vi "u(t)L_test_7.vi"(6 "enable":bool, 7 "Desire Velosity":dbl(slide) scale=-10.0..10.0, 8 "Kd":dbl, 9 "Ki":dbl, 10 "Kp":dbl, 11 "Velocity":dbl) -> (2 "u(t)":dbl)   [LabVIEW 2018]
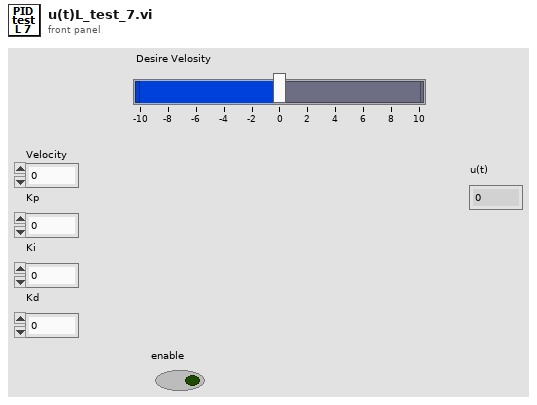
[diagram p1: front panel]
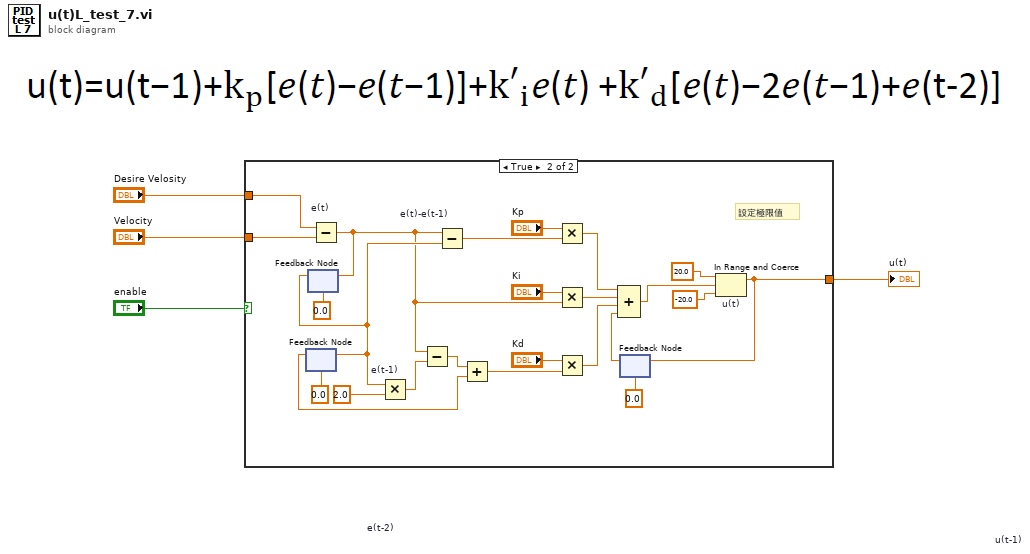
[diagram p0: block diagram]
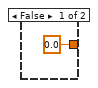
[diagram p2: hidden frame]
diagram:
  n1 = case shown="True" "enable" {
    tunnel: [0.0 ("upper limit") w29] -> w4
    tunnel: "Velocity" -> [_ w11]
    tunnel: "Desire Velosity" -> [_ w10]
    frame False {
    }
    frame True {
      # "設定極限值"
      n2 = feedback #1 "e(t-2)"(0.0) -> (w20:dbl)
      n3 = feedback #2 "e(t-1)"(0.0) -> (w9:dbl)
      n4 = feedback-in #1(w9) -> ()
      n5 = Subtract "e(t)"(x=w10, y=w11) -> (x-y=w8:dbl)
      n6 = feedback-in #2(w8) -> ()
      n7 = Multiply(x=w9, y=2.0) -> (x*y=w18:dbl)
      n8 = Subtract(x=w8, y=w18) -> (x-y=w19:dbl)
      n9 = Subtract "e(t)-e(t-1)"(x=w8, y=w9) -> (x-y=w14:dbl)
      n10 = Add(x=w19, y=w20) -> (x+y=w21:dbl)
      n11 = Multiply(x="Kp", y=w14) -> (x*y=w23:dbl)
      n12 = Multiply(x="Ki", y=w8) -> (x*y=w24:dbl)
      n13 = Multiply(x="Kd", y=w21) -> (x*y=w25:dbl)
      n14 = feedback #3 "u(t-1)"(0.0) -> (w26:dbl)
      n15 = Compound Arithmetic op=ADD(w23, w24, w25, w26) -> (w28:dbl)
      n16 = In Range and Coerce "u(t)"(upper limit=20.0, x=w28, lower limit=-20.0 ("y")) -> (coerced(x)=w29:dbl)  [unwired: 1 out]
      n17 = feedback-in #3(w29) -> ()
    }
  }
  "u(t)" <- w4
